vi "Actor Core.vi"(8 "error in":errorcluster, 11 "IController In":refnum<class "IController.lvclass">) -> (0 "error out":errorcluster, 3 "Actor out":refnum<class "Actor.lvclass">)   [LabVIEW 2015, in "IController.lvlib" / "IController.lvclass"]
doc: "(<B>Filename</B>: Actor Framework.lvlib:Actor.lvclass:Actor Core.vi)\n\nReceives messages to the actor, reacts to them, and initiates any error handling that may shut the actor down.\n\nDescendant classes may override this VI to append parallel tasks for the actor to complete while it handles messages. Overrides use the Call Parent Method node."
uses:
  IController.lvclass
  <vilib>/ActorFramework/Actor/Actor.lvclass
  <vilib>/ActorFramework/Actor/Actor.lvclass/Actor.ctl
  <vilib>/ActorFramework/Message Enqueuer/Message Enqueuer.lvclass/Message Enqueuer.ctl
  <vilib>/ActorFramework/Message Enqueuer/Init from Existing Queue.vi
  <vilib>/ActorFramework/Message Enqueuer/Message Enqueuer.lvclass
  IViewManager/IViewManager/IViewManager.lvclass
  AutoRegistration/ActorAutoRegistration/ActorAutoRegistration.lvclass
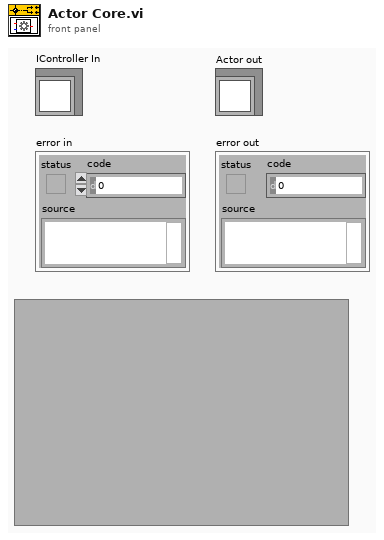
[diagram p1: front panel]
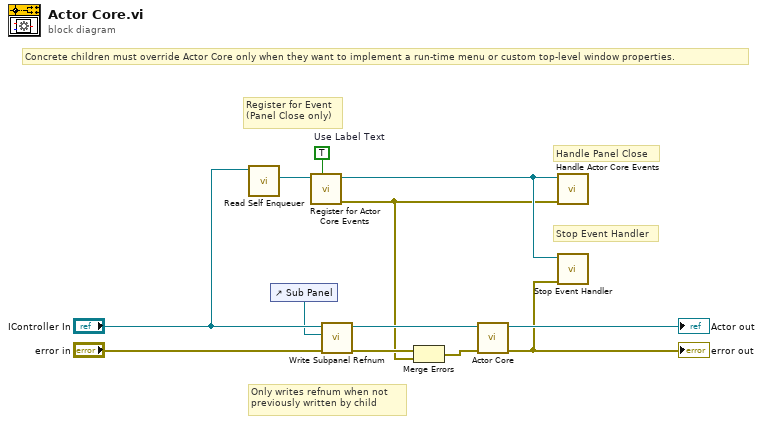
[diagram p0: block diagram]
diagram:
  w3 = TRUE  # Use Label Text
  # "Register for Event\n(Panel Close only)"
  # "Stop Event Handler"
  # "Handle Panel Close"
  # "Only writes refnum when not\npreviously written by child"
  # "Concrete children must override Actor Core only when they want to implement a run-time menu or custom top-level window properties."
  n1 = call <vilib>:"Read Self Enqueuer.vi"("Actor"="IController In") -> ("Self Enqueuer"=w2:refnum<class "Message Enqueuer.lvclass">)  [unwired: 10 in]
  n2 = control-ref of="Sub Panel"() -> (w4:refnum<vi>)
  n3 = call "Register for Actor Core Events.vi"("Use Label Text (F=Use Caption)"=w3, "Actor Enqueuer"=w2) -> ("error out"=w5:errorcluster, "ActorAutoRegistration Out"=w9:refnum<class "ActorAutoRegistration.lvclass">)  [unwired: 8 in]
  n4 = call "Write Subpanel Refnum.vi"("error in (no error)"="error in", "SubPnl Refnum"=w4, "IController In"="IController In") -> ("error out"=w8:errorcluster, "IController Out"=w11:refnum<class "IController.lvclass">)  [unwired: 7 in]
  n5 = Merge Errors(w8, w5) -> (w6:errorcluster)
  n6 = call-parent "Actor Core.vi"("error in"=w6, "IViewable In"=w11) -> ("error out"=w7:errorcluster, "Actor out"=→"Actor out":refnum<class "Actor.lvclass">)  [unwired: 8 in]
  "error out" <- w7
  n7 = call-dynamic "Handle Actor Core Events.vi"("error in (no error)"=w5, "ActorAutoRegistration in"=w9) -> ()  [unwired: 9 in, 1 out]
  n8 = call-dynamic "Stop Event Handler.vi"("error in (no error)"=w7, "ActorAutoRegistration in"=w9) -> ()  [unwired: 9 in, 1 out]
